vi "xiUtils - Cursor Set - Busy.vi"(8 "error in (no error)":errorcluster, 11 "VI reference (Top Level VI)":refnum<vi>) -> (0 "error out":errorcluster, 3 "VI reference (Top Level VI) Out":refnum<vi>)   [LabVIEW 2018]
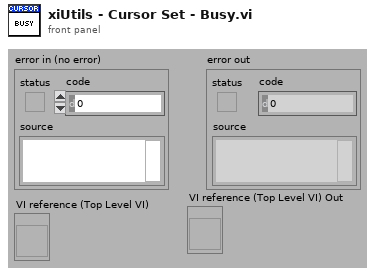
[diagram p1: front panel]
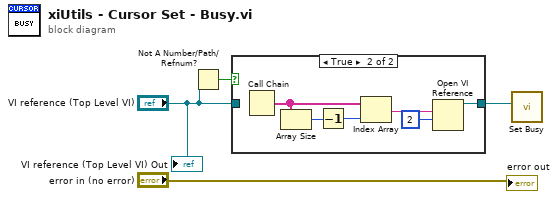
[diagram p0: block diagram]
diagram:
  n1 = Not A Number/Path/Refnum?(number/path/refnum="VI reference (Top Level VI)") -> (NaN/Path/Refnum?=w3:bool)
  n2 = case shown="True" w3 {
    tunnel: "VI reference (Top Level VI)" -> [w5 _]
    tunnel: [w5 w6] -> w1
    frame False {
    }
    frame True {
      n3 = Call Chain() -> (call chain=w10:string[])
      n4 = Array Size(array=w10) -> (size(s)=w9:i32)
      n5 = Decrement(x=w9) -> (x-1=w11:i32)
      n6 = Index Array(array=w10, index=w11) -> (element=w7:string)
      n7 = Open VI Reference(vi path=w7, options=2 ("0x02 =>\nOpen Templates for Editing.  If called by a template, then need template reference.")) -> (vi reference=w6:refnum<vi>)  [unwired: 4 in, 1 out]
    }
  }
  n8 = call <vilib>:"Set Busy.vi"("VI reference (current VI)"=w1) -> ()  [unwired: 9 in, 2 out]
  "error out" <- "error in (no error)"
  "VI reference (Top Level VI) Out" <- "VI reference (Top Level VI)"
